vi "Main.vi"(0 "Path":path, 5 "Stop":bool, 7 "Access":enum16{"read/write", "read-only", "write-only"}(ring), 11 "error in":errorcluster) -> (15 "error out":errorcluster)   [LabVIEW 2020, in "Custom Sort Function.lvlib"]
doc: "This system is used to get paths from the user and then sorts the path in reverse lexicographic order and gives us data like size and the number of items based on the path if it is a file or folder."
uses:
  Libraries/Custom Sort Function.lvlib
panel:
  in  "Store":bool
  out "Description":string[][](table)
  # "CUSTOM SORT PATHS"
  # "INSTRUCTIONS:\n1. Set the way in which you need to get file data.\n2. Then select the file you need to sort.\n3. Then the sorted files with data will be \ndisplayed in the description table.\n4. To get the sorted files with data as a file\nyou can press the store data button to store\nthe data locally."
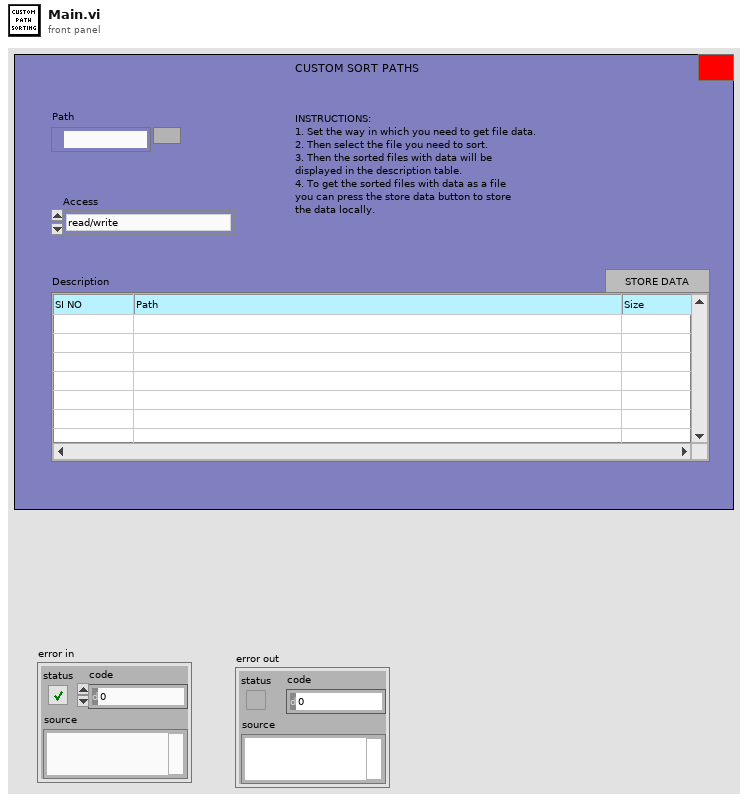
[diagram p1: front panel]
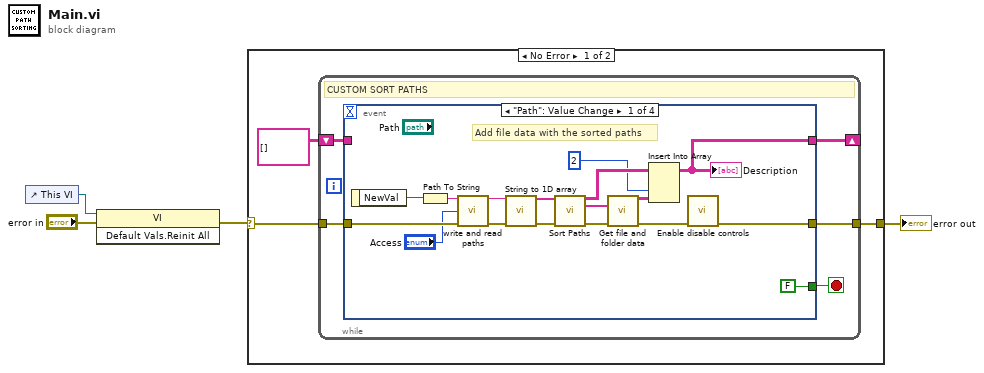
[diagram p0: block diagram]
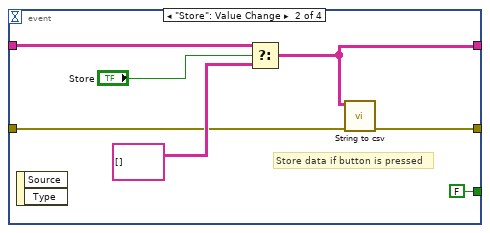
[diagram p2: hidden frame]
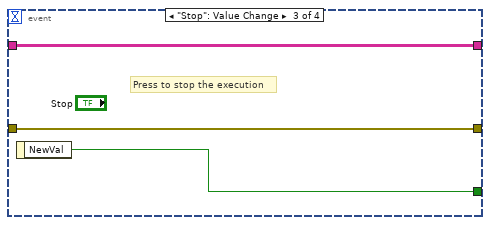
[diagram p3: hidden frame]
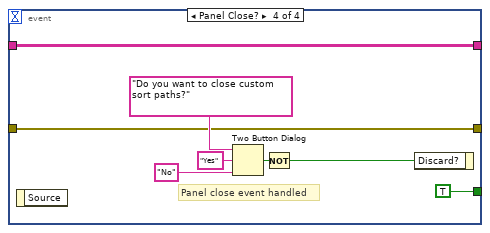
[diagram p4: hidden frame]
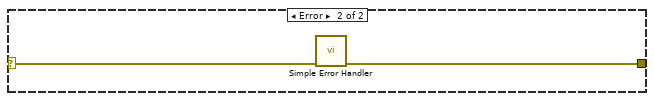
[diagram p5: hidden frame]
diagram:
  n1 = control-ref of="This VI"() -> (w1:refnum<vi>)
  n2 = invoke class="VI" method="Default Vals.Reinit All"(reference=w1, error in="error in") -> (error out=w3:errorcluster)  [unwired: 1 in, 2 out]
  n3 = case shown="No Error" w3 {
    selector: w3 -> [w6 w49]
    tunnel: [w7 w48] -> w4
    frame No Error {
      n4 = while {
        tunnel: [w11] -> w7
        tunnel: w6 -> [w10]
        shift-right: [w9] -> _
        shift-left: string[][] [] ("Table data") -> [w8]
        stop <- w12 stop-if-true
        # "CUSTOM SORT PATHS"
        n5 = event shown="[0] \"Path\": Value Change" {
          selector: _ -> [_ _ _ _]
          dyn-events: _ -> [_ _ _ _]
          timeout: _ -> [_ _ _ _]
          tunnel: [FALSE ("NewVal") FALSE ("NewVal") w39 TRUE ("NewVal")] -> w12
          tunnel: [w18 w32 w38 w41] -> w11
          tunnel: w10 -> [w27 w33 w38 w41]
          tunnel: [w16 w31 w37 w40] -> w9
          tunnel: w8 -> [_ w35 w37 w40]
          event "Path": Value Change {
            # "Add file data with the sorted paths"
            n6 = event-data() -> ("NewVal"=w14:path)  [unwired: 1 in]
            n7 = Path To String(path=w14) -> (string=w24:string)
            n8 = call "write and read paths.vi"("Path"=w24, "Access"="Access", "error in"=w27) -> ("Readed paths"=w26:string, "error out"=w29:errorcluster)  [unwired: 11 in]
            n9 = call "String to 1D array.vi"("Readed paths"=w26, "error in"=w29) -> ("string array"=w25:string[], "error out"=w28:errorcluster)  [unwired: 12 in]
            n10 = call "Sort Paths.vi"("unsorted array"=w25, "error in"=w28) -> ("Table data"=w21:string[][], "sorted array"=w17:string[], "error out"=w22:errorcluster)  [unwired: 11 in]
            n11 = call "Get file and folder data.vi"("Sorted string path"=w17, "Error in"=w22) -> ("file/folder data"=w20:string[][], "Error out"=w15:errorcluster)  [unwired: 12 in]
            n12 = Insert Into Array(array=w21, index (col)=2 ("disabled index (col)"), new element=w20) -> (w16:string[][])  [unwired: 1 in]
            "Description" <- w16
            n13 = call "Enable disable controls.vi"("Error in"=w15) -> ("Error out"=w18:errorcluster)  [unwired: 14 in]
          }
          event "Store": Value Change {
            # "Store data if button is pressed"
            n14 = event-data() -> ()  [unwired: 1 in, 2 out]
            n15 = Select(t=w35, s="Store", f=string[][] []) -> (s? t:f=w31:string[][])
            n16 = call "String to csv.vi"("File data"=w31, "error in"=w33) -> ("error out"=w32:errorcluster)  [unwired: 13 in]
          }
          event "Stop": Value Change {
            # "Press to stop the execution"
            n17 = event-data() -> ("NewVal"=w39:bool)  [unwired: 1 in]
          }
          event Panel Close? {
            # "Panel close event handled"
            n18 = event-data() -> ()  [unwired: 1 in, 1 out]
            n19 = Two Button Dialog(message="Do you want to close custom sort paths?", 1:"No" ("F button name (\"Cancel\")"), 2:"Yes" ("T button name (\"OK\")")) -> (T button?=w46:bool)
            n20 = Not(x=w46) -> (.not. x?=w47:bool)
            n21 = event-data("Discard?"=w47) -> ()  [unwired: 1 in, 1 out]
          }
        }
      }
    }
    frame Error {
      n22 = call <vilib>:"Simple Error Handler.vi"("error in (no error)"=w49) -> ("error out"=w48:errorcluster)  [unwired: 4 in, 4 out]
    }
  }
  "error out" <- w4
